vi "PR_Update_glue_data .vi"(7 "glue_data_id":string, 8 "error in (no error)":errorcluster, 10 "barcode":string="05050505", 11 "DBlink":string="Driver={ODBC Driver 17 for SQL Server};Server=localhost\\SQLEXPRESS;Database=ZDX201;UID=labview;PWD=Dsa@54137926") -> (0 "error out":errorcluster)   [LabVIEW 2019]
uses:
  <vilib>/addons/database/Connection.llb/DB Tools Open Connec (String).vi
  <vilib>/addons/database/NI_Database_API.lvlib
panel:
  out "Command":string="WHERE [barcode]='05050505' and [position]='B'\nand assemble_time is not null"
  in  "columns":string[](array[string])=["done_time", "update_time", "glue_data_id"]
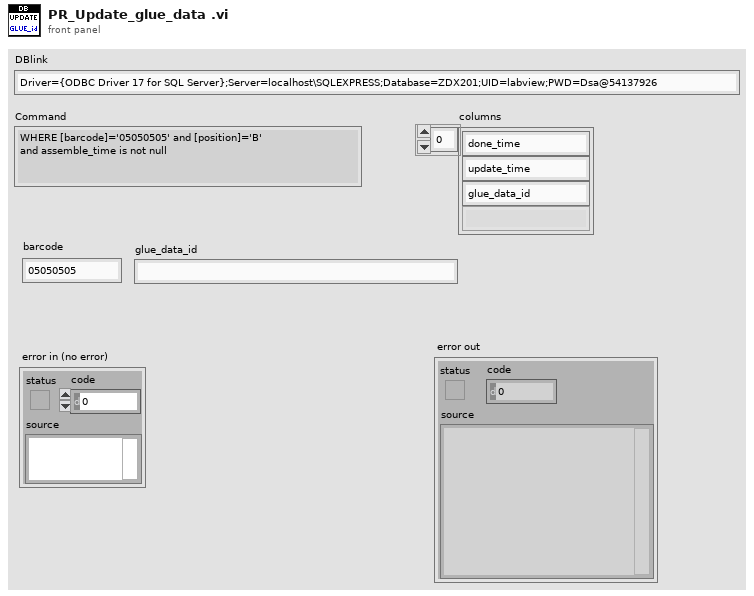
[diagram p1: front panel]
types:
  T1 = cluster{"done_time":timestamp, "update_time":timestamp, "glue_data_id":string}
  T2 = typedef "NI_Database_API.lvlib/Conn ObjectReference.ctl" = refnum<k1>
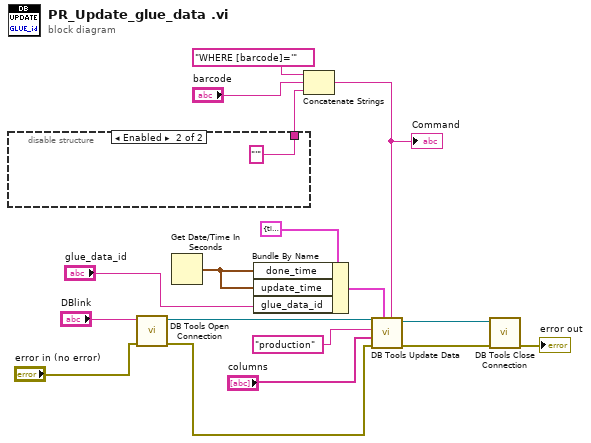
[diagram p0: block diagram]
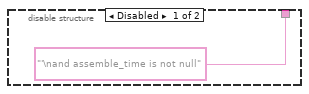
[diagram p2: hidden frame]
diagram:
  n1 = disable-structure shown="Enabled" {
    disable-tunnel: ["'\nand assemble_time is not null" ("string") "'"] -> w5
    frame Disabled {
    }
    frame Enabled {
    }
  }
  n2 = call-poly <vilib>:"DB Tools Open Connection.vi"("error in (no error)"="error in (no error)", "connection information"="DBlink") -> ("error out"=w15:errorcluster, "connection reference"=w13:T2)  [unwired: 6 in]
  n3 = Get Date/Time In Seconds() -> (seconds since 1Jan1904=w3:timestamp)
  n4 = Bundle By Name(cluster=T1 {"done_time"=timestamp(0 s since 1904-01-01), "update_time"=timestamp(0 s since 1904-01-01), "glue_data_id"=""}, "done_time"=w3, "update_time"=w3, "glue_data_id"="glue_data_id") -> (w2:T1)
  n5 = Concatenate Strings("WHERE [barcode]='", "barcode", w5) -> (w7:string)
  "Command" <- w7
  n6 = call <vilib>:"DB Tools Update Data.vi"("condition"=w7, "data"=w2, "error in (no error)"=w15, "columns"="columns", "table"="production", "connection reference"=w13) -> ("error out"=w16:errorcluster, "connection reference out"=w14:T2)  [unwired: 4 in]
  n7 = call <vilib>:"DB Tools Close Connection.vi"("error in (no error)"=w16, "connection reference"=w14) -> ("error out"=→"error out":errorcluster)  [unwired: 5 in]
